vi "Read netCDF Metadata.vi"(8 "error in (no error)":errorcluster, 9 "key":string, 10 "file path":path, 11 "Refnum in":refnum<k35>) -> (0 "error out":errorcluster, 2 "Value":string, 3 "Refnum out":refnum<k35>)   [LabVIEW 2019]
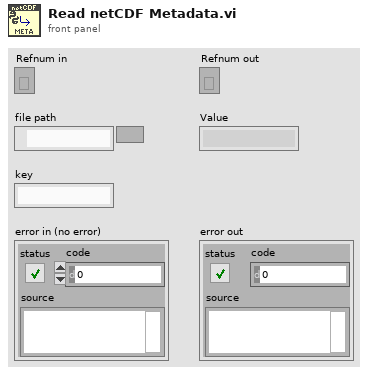
[diagram p1: front panel]
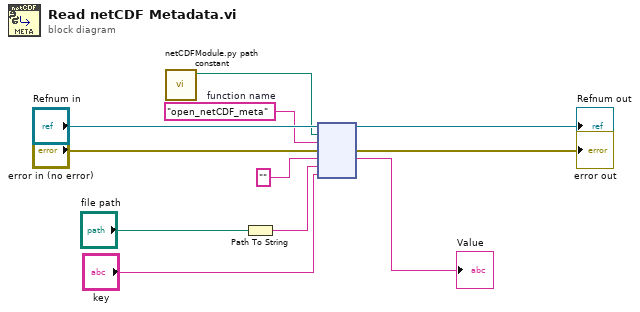
[diagram p0: block diagram]
diagram:
  w5 = "open_netCDF_meta"  # function name
  n1 = call "netCDFModule.py path constant.vi"() -> ("appended path"=w1:path)  [unwired: 11 in]
  n2 = Path To String(path="file path") -> (string=w10:string)
  n3 = node("Refnum in", w1, w5, "error in (no error)", "", w10, "key") -> (→"Refnum out":refnum<k35>, →"error out":errorcluster, →"Value":string)  [unwired: 2 in, 2 out]
